vi "Blend.vi"(7 "Source Name in":string, 8 "error in (no error)":errorcluster, 9 "Source Enqueuer":refnum<class "Message Enqueuer.lvclass">, 10 "Sample to Blend in":refnum<class "Sample.lvclass">, 11 "Sample Line in":refnum<class "Sample Line.lvclass">) -> (0 "error out":errorcluster, 2 "Source Name":string, 3 "Sample Line out":refnum<class "Sample Line.lvclass">)   [LabVIEW 2015, in "cRIO-Carbondioxide.lvlib" / "CO2-Actor.lvlib" / "Sample Line.lvclass"]
uses:
  Sample Line.lvclass
  subs/Sample/Sample.lvclass
  <vilib>/ActorFramework/Message Enqueuer/Message Enqueuer.lvclass
  CO2 Actor/CO2 Actor.lvclass
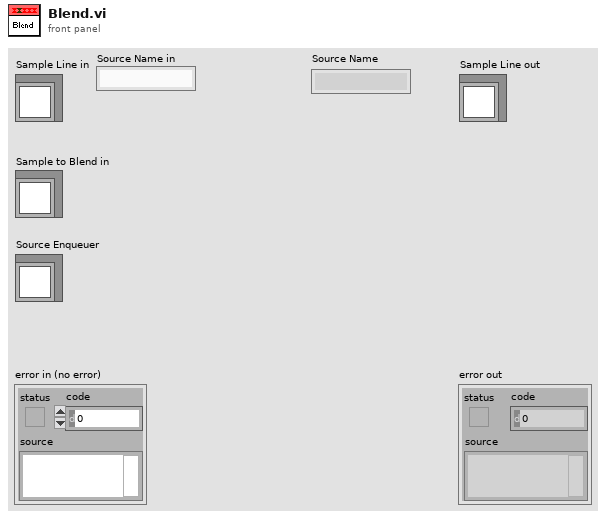
[diagram p1: front panel]
types:
  T1 = typedef "Sample Line State Enumerator.ctl" = enum16{"All lines closed", "Sample line 1.", "Sample line 2.", "Sample line 3.", "Sample line 4.", "Sample line 5.", "Out of range"}
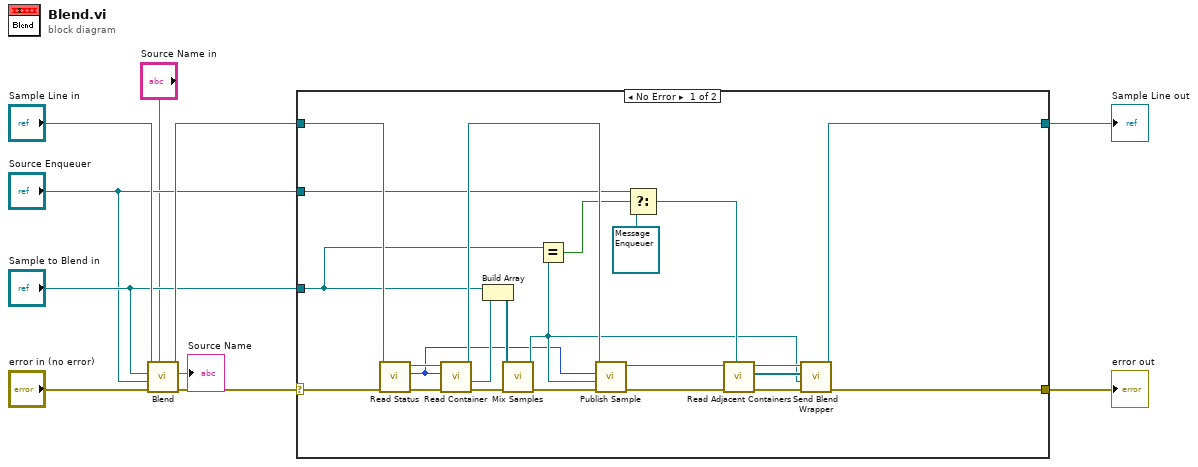
[diagram p0: block diagram]
diagram:
  n1 = call-parent "Blend.vi"("Source Name in"="Source Name in", "error in (no error)"="error in (no error)", "Source Enqueuer"="Source Enqueuer", "Sample to Blend in"="Sample to Blend in", "CO2 Actor in"="Sample Line in") -> ("error out"=w7:errorcluster, "Source Name"=→"Source Name":string, "CO2 Actor out"=w5:refnum<class "Sample Line.lvclass">)  [unwired: 4 in]
  n2 = case shown="No Error" w7 {
    selector: w7 -> [w33 w35]
    tunnel: "Source Enqueuer" -> [w22 _]
    tunnel: "Sample to Blend in" -> [w14 _]
    tunnel: w5 -> [w27 w34]
    tunnel: [w15 w35] -> w9
    tunnel: [w16 w34] -> w10
    frame No Error {
      n3 = call "Read Status.vi"("error in (no error)"=w33, "Sample Line in"=w27) -> ("error out"=w28:errorcluster, "Status"=w11:T1, "Sample Line out"=w29:refnum<class "Sample Line.lvclass">)  [unwired: 7 in]
      n4 = call "Read Container.vi"("error in (no error)"=w28, "Sample Line (All Closed)"=w11, "Sample Line in"=w29) -> ("error out"=w32:errorcluster, "Sample"=w31:refnum<class "Sample.lvclass">, "Sample Line out"=w25:refnum<class "Sample Line.lvclass">)  [unwired: 5 in, 1 out]
      n5 = Build Array(w14, w31) -> (w30:refnum<class "Sample.lvclass">[])
      n6 = call "Mix Samples.vi"("error in (no error)"=w32, "Samples In"=w30) -> ("error out"=w26:errorcluster, "Sample out"=w13:refnum<class "Sample.lvclass">)  [unwired: 6 in, 2 out]
      n7 = Equal?(x=w14, y=w13) -> (x = y?=w12:bool)
      n8 = call "Publish Sample.vi"("error in (no error)"=w26, "Sample"=w13, "Sample Line (All Closed)"=w11, "Sample Line in"=w25) -> ("error out"=w23:errorcluster, "Sample Line in 2"=w24:refnum<class "Sample Line.lvclass">)  [unwired: 6 in]
      n9 = Select(t=w22, s=w12, f=refnum<class "Message Enqueuer.lvclass"> refnum) -> (s? t:f=w21:refnum<class "Message Enqueuer.lvclass">)
      n10 = call "Read Adjacent Containers.vi"("Exclude Source"=w21, "error in (no error)"=w23, "Sample Line in"=w24) -> ("error out"=w19:errorcluster, "Adjacent Containers"=w17:refnum<class "Message Enqueuer.lvclass">[], "Sample Line out"=w18:refnum<class "Sample Line.lvclass">)  [unwired: 6 in]
      n11 = call-dynamic "Send Blend Wrapper.vi"("error in (no error)"=w19, "Sample to Blend"=w13, "Send to"=w17, "CO2 Actor in"=w18) -> ("error out"=w15:errorcluster, "CO2 Actor out"=w16:refnum<class "Sample Line.lvclass">)  [unwired: 6 in]
    }
    frame Error {
    }
  }
  "error out" <- w9
  "Sample Line out" <- w10
